vi "Fix Route.vi"(1 "Route":string) -> (0 "Proper Route":string)   [LabVIEW 2023, in "Server.lvclass"]
uses:
  Server.lvclass
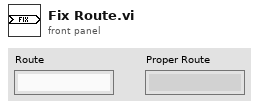
[diagram p1: front panel]
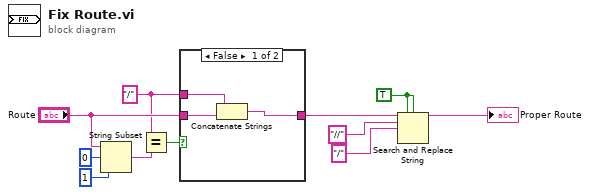
[diagram p0: block diagram]
diagram:
  w1 = TRUE
  w6 = "/" ("y")
  n1 = String Subset(string="Route", offset (0)=0, length (rest)=1 ("length (rest)")) -> (substring=w9:string)
  n2 = Equal?(x=w6, y=w9) -> (x = y?=w8:bool)
  n3 = case shown="False" w8 {
    tunnel: [w12 w15] -> w5
    tunnel: "Route" -> [w14 w15]
    tunnel: w6 -> [w13 _]
    frame False {
      n4 = Concatenate Strings(w13, w14) -> (w12:string)
    }
    frame True {
    }
  }
  n5 = Search and Replace String(replace all?=w1, case sensitive?=w1, input string=w5, search string="//" ("y"), replace string="/" ("y")) -> (result string=→"Proper Route":string)  [unwired: 3 in, 3 out]
